vi "disdrometer_dataparse_2020_05_05.vi"(11 "Poll Response":string) -> (4 "Complete Dataset":string[](array[string]), 8 "output cluster":T2, 10 "Spectrum Data":dbl[](array[numeric]), 14 "DisdromStatus":T1={"Laser"=TRUE, "Signal"=TRUE, "LaserTemp_Analog"=TRUE, "LaserTemp_Digital"=TRUE, "LaserCurrent_Analog"=TRUE, "LaserCurrent_Digital"=TRUE, "SensorSupply"=TRUE, "HeatLaserHead"=TRUE, "HeatReceiverHead"=TRUE, "TempSensor"=TRUE, "HeatSupply"=TRUE, "HeatHousing"=TRUE, "HeatHeads"=TRUE, "HeatCarriers"=TRUE, "OutputLaserPower"=TRUE, "Checksum"=TRUE, "StatusInt"=0})   [LabVIEW 2018]
doc: "Given a poll response from the Thies Clima disdrometer, deciphers the response string into arrays. Available ouputs include the complete dataset array, or subarrays seperated into general data, spectrum data, and debug data."
uses:
  Epimedia_Connex_Source/HDF5/DisdromterSummaryData.ctl
  Disdrometer_Status_Cluster.ctl
panel:
  out "replaced substring":string
  out "ToDisplay":dbl[](array[numeric])
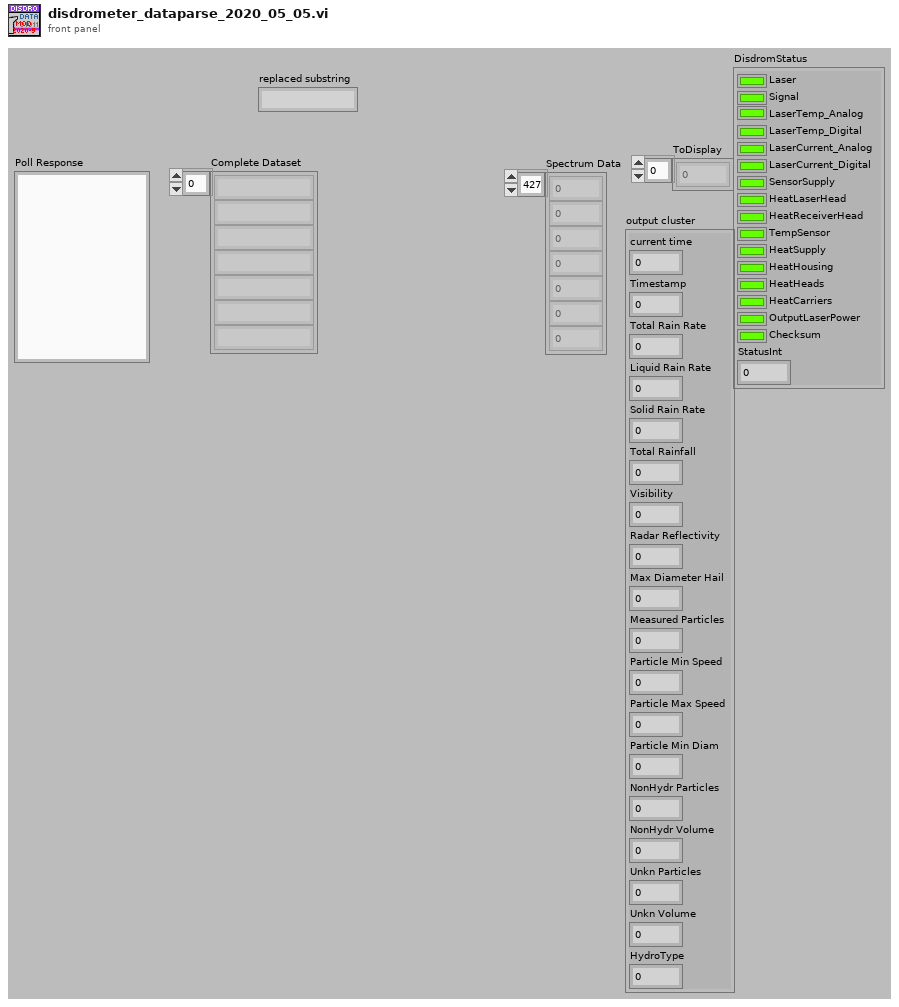
[diagram p1: front panel]
types:
  T1 = typedef "Disdrometer_Status_Cluster.ctl" = cluster{"Laser":bool, "Signal":bool, "LaserTemp_Analog":bool, "LaserTemp_Digital":bool, "LaserCurrent_Analog":bool, "LaserCurrent_Digital":bool, "SensorSupply":bool, "HeatLaserHead":bool, "HeatReceiverHead":bool, "TempSensor":bool, "HeatSupply":bool, "HeatHousing":bool, "HeatHeads":bool, "HeatCarriers":bool, "OutputLaserPower":bool, "Checksum":bool, "StatusInt":u16}
  T2 = typedef "DisdromterSummaryData.ctl" = cluster{"current time":dbl, "Timestamp":dbl, "Total Rain Rate":dbl, "Liquid Rain Rate":dbl, "Solid Rain Rate":dbl, "Total Rainfall":dbl, "Visibility":dbl, "Radar Reflectivity":dbl, "Max Diameter Hail":dbl, "Measured Particles":i32, "Particle Min Speed":i16, "Particle Max Speed":i16, "Particle Min Diam":i16, "NonHydr Particles":i16, "NonHydr Volume":dbl, "Unkn Particles":i16, "Unkn Volume":dbl, "HydroType":i8}
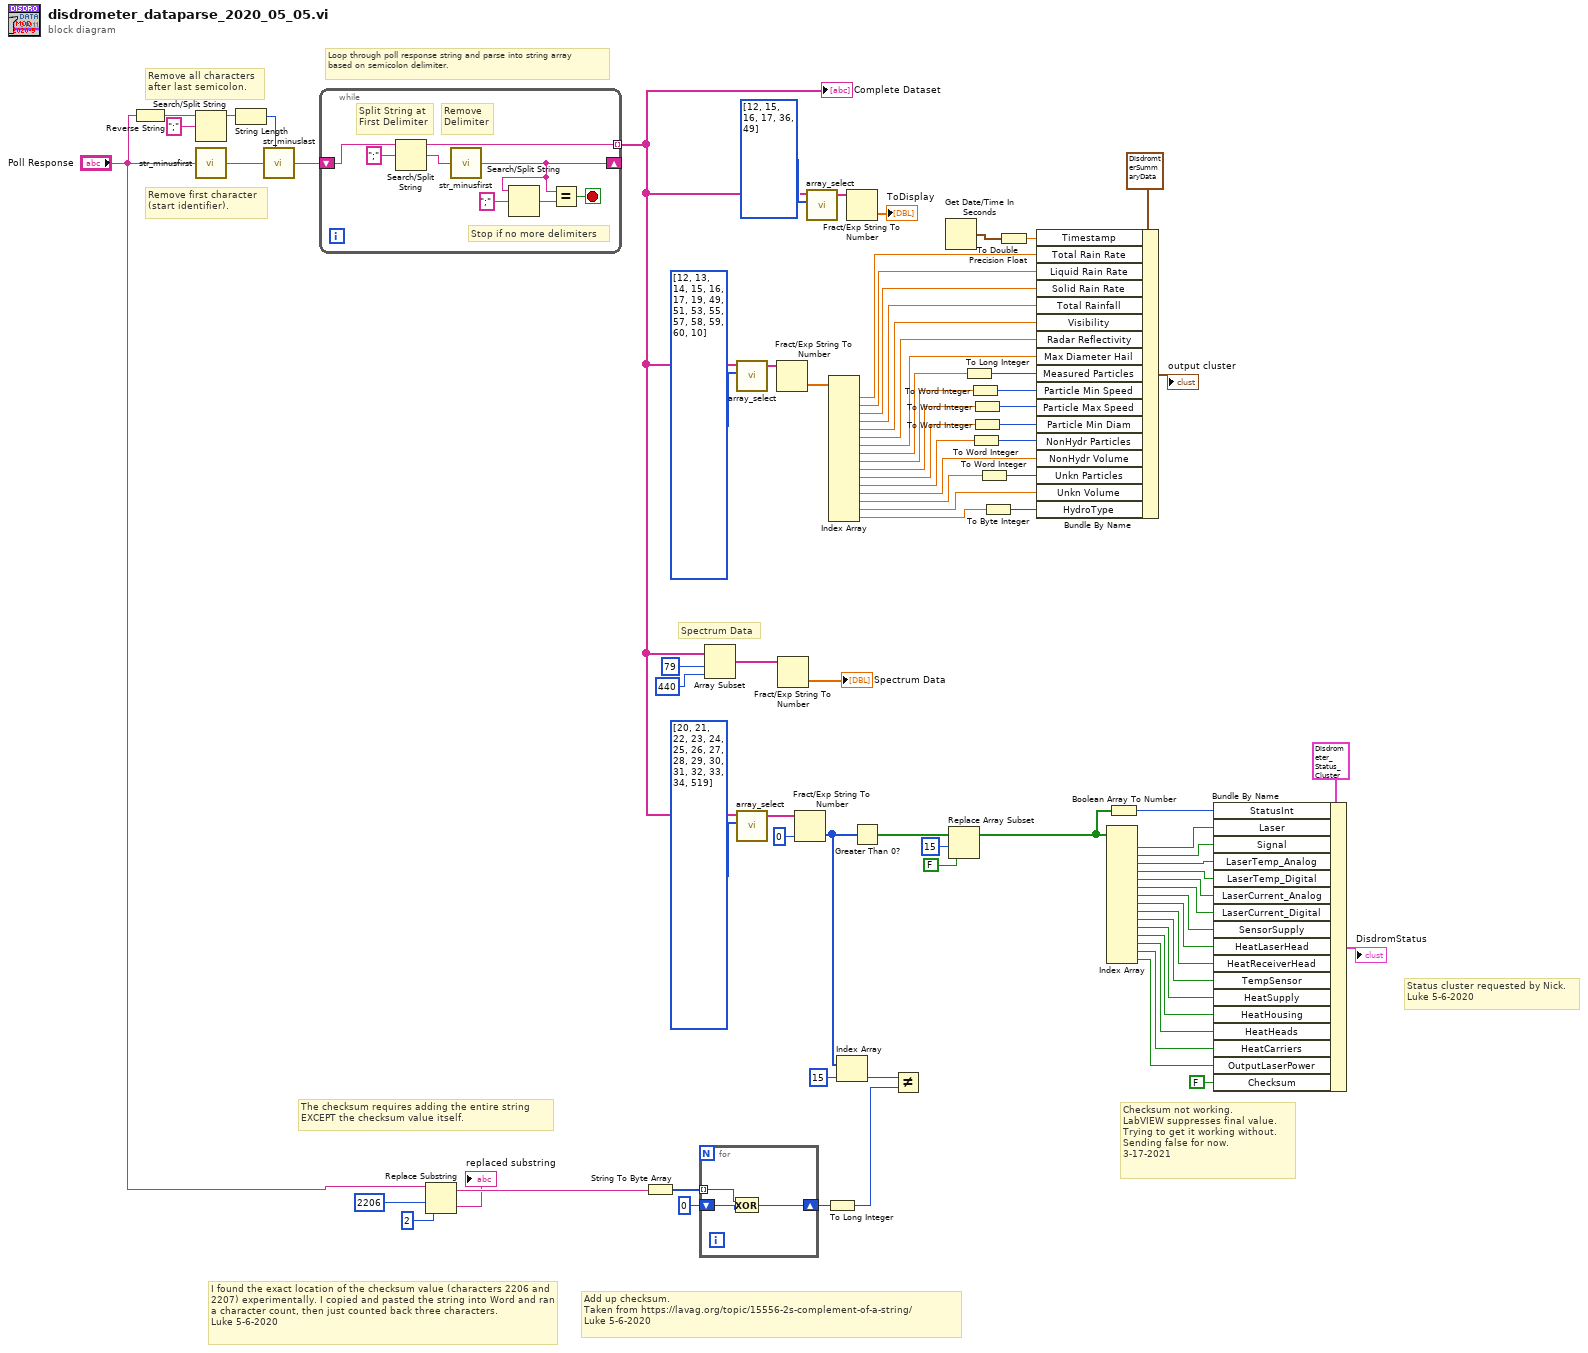
[diagram p0: block diagram]
diagram:
  # "Checksum not working. \nLabVIEW suppresses final value.\nTrying to get it working without.\nSending false for now.\n3-17-2021"
  # "I found the exact location of the checksum value (characters 2206 and 2207) experimentally. I copied and pasted the string into Word and ran a character count, then just counted back three characters.\nLuke 5-6-2020"
  # "The checksum requires adding the entire string \nEXCEPT the checksum value itself."
  # "Status cluster requested by Nick.\nLuke 5-6-2020"
  # "Add up checksum.\nTaken from https://lavag.org/topic/15556-2s-complement-of-a-string/\nLuke 5-6-2020"
  # "Spectrum Data"
  # "Remove all characters\nafter last semicolon."
  # "Remove first character\n(start identifier)."
  # "Loop through poll response string and parse into string array\nbased on semicolon delimiter."
  n1 = Reverse String(1:"Poll Response") -> (0:w79:string)
  n2 = Search/Split String(string=w79, search string/char (-)=";") -> (substring before match=w78:string)  [unwired: 1 in, 2 out]
  n3 = call "str_minusfirst.vi"("String In"="Poll Response") -> ("String Out"=w82:string)  [unwired: 6 in]
  n4 = String Length(string=w78) -> (length=w77:i32)
  n5 = call "str_minuslast.vi"("N"=w77, "String In"=w82) -> ("String Out"=w81:string)  [unwired: 5 in]
  n6 = while {
    tunnel: [w89] -> w39 mode=indexing
    shift-right: [w83] -> _
    shift-left: w81 -> [w88]
    stop <- w87 stop-if-true
    # "Stop if no more delimiters"
    # "Remove\nDelimiter"
    # "Split String at\nFirst Delimiter"
    n7 = Search/Split String(string=w88, search string/char (-)=";") -> (substring before match=w89:string, match + rest of string=w86:string)  [unwired: 1 in, 1 out]
    n8 = call "str_minusfirst.vi"("String In"=w86) -> ("String Out"=w83:string)  [unwired: 6 in]
    n9 = Search/Split String(string=w83, search string/char (-)=";") -> (match + rest of string=w85:string)  [unwired: 1 in, 2 out]
    n10 = Equal?(x=w83, y=w85) -> (x = y?=w87:bool)
  }
  "Complete Dataset" <- w39
  n11 = Replace Substring(2:2 ("length (len. of substring)"), 3:2206 ("offset"), 5:"Poll Response") -> (0:→"replaced substring":string, 1:w11:string)  [unwired: 1 in]
  n12 = String To Byte Array(string=w11) -> (unsigned byte array=w18:u8[])
  n13 = for {
    tunnel: w18 -> [w93] mode=indexing
    shift-right: [w92] -> w16
    shift-left: u8 0 -> [w91]
    n14 = Exclusive Or(1:w91, 2:w93) -> (0:w92:u8)
  }
  n15 = Array Subset(array=w39, index=79, length=440) -> (w57:string[])
  n16 = call "array_select.vi"("Selection"=i32[] [12, 13, 14, 15, 16, 17, 19, 49, 51, 53, 55, 57, 58, 59, 60, 10], "Array In"=w39) -> ("Array Out"=w74:string[])  [unwired: 9 in]
  n17 = call "array_select.vi"("Selection"=i32[] [20, 21, 22, 23, 24, 25, 26, 27, 28, 29, 30, 31, 32, 33, 34, 519], "Array In"=w39) -> ("Array Out"=w40:string[])  [unwired: 9 in]
  n18 = Fract/Exp String To Number(string=w74) -> (number=w69:dbl[])  [unwired: 3 in, 1 out]
  n19 = Fract/Exp String To Number(string=w57) -> (number=→"Spectrum Data":dbl[])  [unwired: 3 in, 1 out]
  n20 = Fract/Exp String To Number(string=w40, default (0 dbl)=0 ("default (0 DBL)")) -> (number=w21:i32[])  [unwired: 2 in, 1 out]
  n21 = call "array_select.vi"("Selection"=i32[] [12, 15, 16, 17, 36, 49], "Array In"=w39) -> ("Array Out"=w71:string[])  [unwired: 9 in]
  n22 = To Long Integer(number=w16) -> (32bit integer=w15:i32)
  n23 = Index Array(array=w69) -> (element #1=w68:dbl, element #2=w67:dbl, element #3=w66:dbl, element #4=w65:dbl, element #5=w64:dbl, element #6=w63:dbl, element #7=w62:dbl, element #8=w61:dbl, element #9=w53:dbl, element #10=w52:dbl, element #11=w51:dbl, element #12=w50:dbl, element #13=w60:dbl, element #14=w44:dbl, element #15=w59:dbl, element #16=w45:dbl)  [unwired: 16 in]
  n24 = Index Array(array=w21, index=15) -> (element=w19:i32)
  n25 = Fract/Exp String To Number(string=w71) -> (number=→"ToDisplay":dbl[])  [unwired: 3 in, 1 out]
  n26 = Greater Than 0?(x=w21) -> (x > 0?=w8:bool[])
  n27 = Not Equal?(x=w19, y=w15) -> ()  [unwired: 1 out]
  n28 = Get Date/Time In Seconds() -> (seconds since 1Jan1904=w1:timestamp)
  n29 = Replace Array Subset(array=w8, new element=FALSE ("new element/subarray"), index=15) -> (w5:bool[])
  n30 = To Long Integer(number=w61) -> (32bit integer=w54:i32)
  n31 = To Word Integer(number=w53) -> (16bit integer=w46:i16)
  n32 = To Word Integer(number=w50) -> (16bit integer=w49:i16)
  n33 = To Word Integer(number=w52) -> (16bit integer=w47:i16)
  n34 = To Word Integer(number=w51) -> (16bit integer=w48:i16)
  n35 = To Word Integer(number=w44) -> (16bit integer=w43:i16)
  n36 = To Byte Integer(number=w45) -> (8bit integer=w42:i8)
  n37 = To Double Precision Float(number=w1) -> (double precision float=w2:dbl)
  n38 = Bundle By Name(cluster=T2 {"current time"=0.0, "Timestamp"=0.0, "Total Rain Rate"=0.0, "Liquid Rain Rate"=0.0, "Solid Rain Rate"=0.0, "Total Rainfall"=0.0, "Visibility"=0.0, "Radar Reflectivity"=0.0, "Max Diameter Hail"=0.0, "Measured Particles"=0, "Particle Min Speed"=0, "Particle Max Speed"=0, "Particle Min Diam"=0, "NonHydr Particles"=0, "NonHydr Volume"=0.0, "Unkn Particles"=0, "Unkn Volume"=0.0, "HydroType"=0} ("DisdromSummary"), "Timestamp"=w2, "Total Rain Rate"=w68, "Liquid Rain Rate"=w67, "Solid Rain Rate"=w66, "Total Rainfall"=w65, "Visibility"=w64, "Radar Reflectivity"=w63, "Max Diameter Hail"=w62, "Measured Particles"=w54, "Particle Min Speed"=w46, "Particle Max Speed"=w47, "Particle Min Diam"=w48, "NonHydr Particles"=w49, "NonHydr Volume"=w60, "Unkn Particles"=w43, "Unkn Volume"=w59, "HydroType"=w42) -> (→"output cluster":T2)
  n39 = Index Array(array=w5) -> (element #1=w36:bool, element #2=w35:bool, element #3=w34:bool, element #4=w33:bool, element #5=w32:bool, element #6=w31:bool, element #7=w30:bool, element #8=w29:bool, element #9=w28:bool, element #10=w27:bool, element #11=w26:bool, element #12=w25:bool, element #13=w24:bool, element #14=w23:bool, element #15=w22:bool)  [unwired: 15 in]
  n40 = Boolean Array To Number(Boolean array=w5) -> (number=w7:u16)
  n41 = Bundle By Name(cluster=T1 {"Laser"=TRUE, "Signal"=TRUE, "LaserTemp_Analog"=TRUE, "LaserTemp_Digital"=TRUE, "LaserCurrent_Analog"=TRUE, "LaserCurrent_Digital"=TRUE, "SensorSupply"=TRUE, "HeatLaserHead"=TRUE, "HeatReceiverHead"=TRUE, "TempSensor"=TRUE, "HeatSupply"=TRUE, "HeatHousing"=TRUE, "HeatHeads"=TRUE, "HeatCarriers"=TRUE, "OutputLaserPower"=TRUE, "Checksum"=TRUE, "StatusInt"=0}, "StatusInt"=w7, "Laser"=w36, "Signal"=w35, "LaserTemp_Analog"=w34, "LaserTemp_Digital"=w33, "LaserCurrent_Analog"=w32, "LaserCurrent_Digital"=w31, "SensorSupply"=w30, "HeatLaserHead"=w29, "HeatReceiverHead"=w28, "TempSensor"=w27, "HeatSupply"=w26, "HeatHousing"=w25, "HeatHeads"=w24, "HeatCarriers"=w23, "OutputLaserPower"=w22, "Checksum"=FALSE) -> (→"DisdromStatus":T1)
